vi "Untitled 2 (SubVI).vi"(8 "error in (no error)":errorcluster, 10 "Horizontal Scrollbar Visibility":T1(ring), 11 "Pane in":refnum<vi>) -> (0 "error out":errorcluster, 3 "Pane in 2":refnum<vi>)   [LabVIEW 2015]
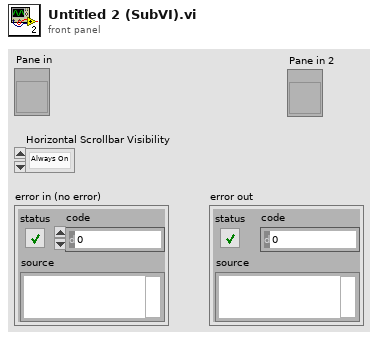
[diagram p1: front panel]
types:
  T1 = enum16{"Always On", "Always Off", "Off While Running"}
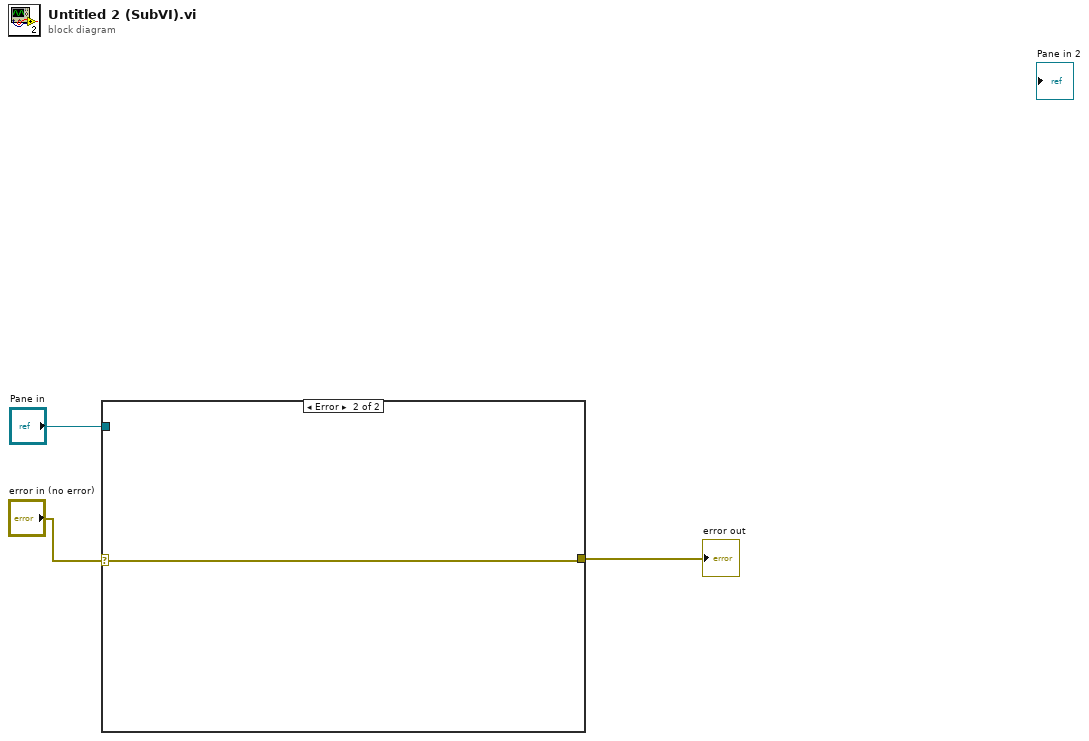
[diagram p0: block diagram]
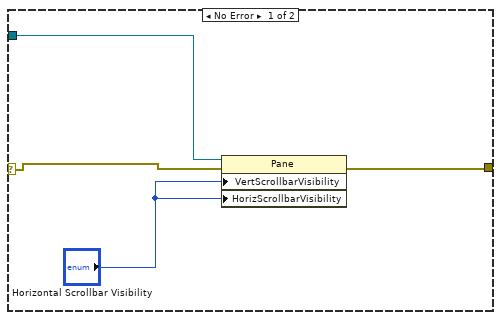
[diagram p2: hidden frame]
diagram:
  n1 = case shown="Error" "error in (no error)" {
    selector: "error in (no error)" -> [w4 w8]
    tunnel: [w6 w8] -> w3
    tunnel: "Pane in" -> [w5 _]
    frame No Error {
      n2 = property on="Property Node" class="Pane"(reference=w5, error in=w4, "VertScrollbarVisibility"="Horizontal Scrollbar Visibility", "HorizScrollbarVisibility"="Horizontal Scrollbar Visibility") -> (error out=w6:errorcluster)  [unwired: 1 out]
    }
    frame Error {
    }
  }
  "error out" <- w3
